vi "CJ_ADV.vi"() -> (5 "Plug in titles":string[](array[string]), 7 "Plug in values":string[](array[string]))   [LabVIEW 2010]
uses:
  Controls/Post_Process.ctl
  Globals/Meas_global.vi
  Globals/Plug_in_data_global.vi
panel:
  in  "Case Constant\n(See Context Help)":bool=TRUE
  out "Spectrum":cluster{dbl, dbl, dbl[][]}(graph)
  in  "Approx period":dbl=2.0 format="%.2f"
  in  "End chop":i32
  in  "Start chop":i32
  out "Auto correlation":cluster{dbl, dbl, dbl[]}[](graph)=[{0.2, 0.04, [0.46212378181095987, 0.44544943210747023, 0.39960558861098977, 0.3343117058776894, 0.2633632126098303, 0.21884653665959014, 0.1564325599910705, 0.12187113727101749, 0.06431157992181454, 0.0061376685707129775, -0.05669014852994204, -0.11505485081145915, -0.174459405708325, -0.19680472077091235, -0.2355643441337355, -0.279169576323247, -0.3107773861747396, -0.34177721677867895, -0.32552035787602773, -0.31390078612386346, -0.3141404513979377, -0.3203374677759062, -0.2805277493481923, -0.28030627175161327, -0.24878188504536167, -0.20171526154420918, -0.17478453331117821, -0.1492406112692455, -0.09716915086627186, -0.011036547249165897, 0.011273554688758552, 0.05137612064072646, 0.08633160095444244, 0.16325012318844126, 0.18825734545368525, 0.2399050524128652, 0.27148875410835505, 0.3135098324885922, 0.3339189753369369, 0.3532110595738442, 0.369889458228514, 0.4018515159612758, 0.3407037745996836, 0.3734587832352109, 0.33095796252280335, 0.3130223675527058, 0.28047256007652444, 0.2305017307249458, 0.24409104361634573, 0.22534283311709877, 0.19096120764523986, 0.10889483405727994, 0.06279838820183563, 0.014744937155805955, -0.02875404241397365, -0.02585905719816059, -0.06912125525736, -0.12596797235968518, -0.16959473872415834, -0.19587644981544367, -0.21534151184322906, -0.23255107675816336, -0.22831112695227931, -0.2179940037588913, -0.21577075545502555, -0.23768491590732238, -0.25009985440842564, -0.21883085511678074, -0.14982831467783184, -0.18257249609141823]}, {0.2, 0.04, [0.455531353534939, 0.4047541811650962, 0.3471922482149264, 0.2503699209196126, 0.20135079931123062, 0.11260724349217213, 0.034422569726896945, -0.030285571006114807, -0.11909404419991482, -0.18269038617194974, -0.23796709263127072, -0.2926953340047305, -0.35993422522198565, -0.4128421353811272, -0.45929580276986665, -0.5004541855522154, -0.5152391710086142, -0.51648559321319, -0.5271510882708651, -0.4806134161451423, -0.4850035395287815, -0.4662260004246924, -0.43183224812859133, -0.3975046428001596, -0.32639935049887153, -0.2795320771193606, -0.20861339510620014, -0.13136107527816313, -0.0788014018836706, -0.00855171247713191, 0.0298850880210123, 0.09776334527023417, 0.1785154642333505, 0.24021430276852615, 0.32501027179400727, 0.3418682226217491, 0.38756231445126293, 0.38959926105408205, 0.424467596341874, 0.4477619180529467, 0.4311914530598441, 0.4316664497716769, 0.4294595730219442, 0.4129090596655477, 0.3728855522699742, 0.35098699804248196, 0.3125013768615565, 0.25447334339580563, 0.20324298562375057, 0.166027641267823, 0.09557452943638053, 0.05023082102923798, -0.0032482398578684846, -0.05105953152757626, -0.13062652237796318, -0.19685300112362478, -0.24586301223225085, -0.2846838464872371, -0.3213134567643425, -0.3686474080102875, -0.40647088073256527, -0.4420878010421662, -0.4390774208886359, -0.4702929313038014, -0.4021180460569205, -0.37623488168286134, -0.3275070404289632, -0.3233751790837929, -0.2685900219122207, -0.23859579085375265]}]
  out "Clipped length":i32=524
  out "Time trace":cluster{dbl[], dbl[]}[](graph)
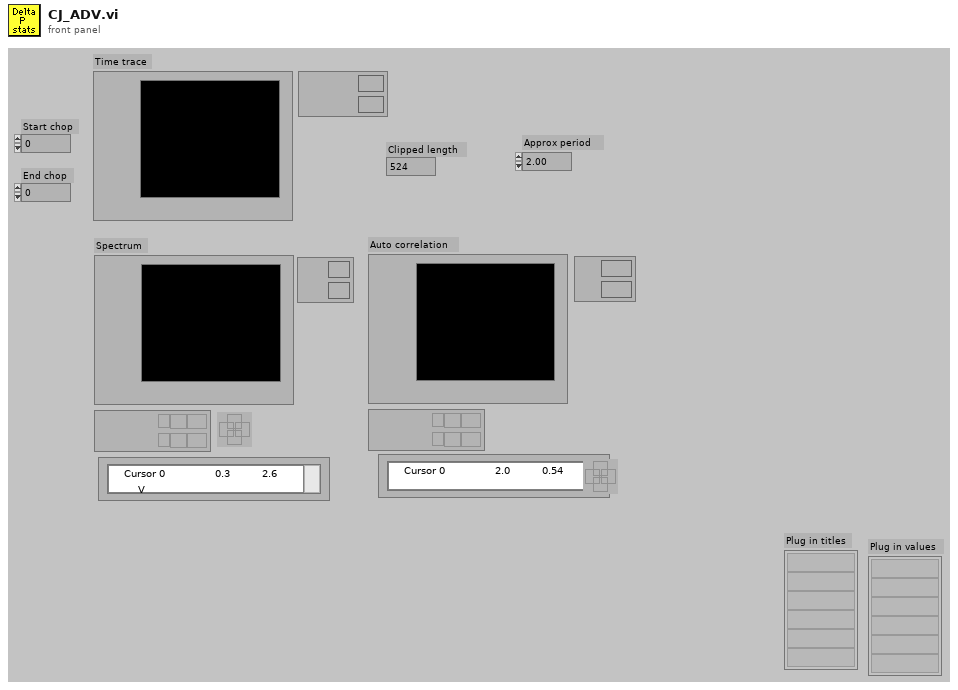
[diagram p1: front panel]
types:
  T1 = typedef "Post_Process.ctl" = enum16{"Take New Data", "Post Process Raw Data File"}
  T2 = typedef "Analysis_info_cluster.ctl" = cluster{"Colour":u32, "Inst type":T3, "Inst name":string, "Symbol":string, "Code name":string, "Extra Info":string, "Inst Array":T4, "Index":i32, "Voltage Index":i32, "Extra Titles":string[], "Extra Values":string[]}
  T3 = typedef "Inst_type.ctl" = enum16{"Propeller anemometer", "Raw voltage", "Pressure Transducer", "Pitot-static tube", "Preston tube", "Hot wire", "Cross wire 1", "Cross wire 2", "Generic Linear", "Generic Polynomial", "Generic BackPoly", "Fast FID", "Thermocouple", "Cold wire", "Pulsed Wire", "LDA Vel", "LDA Tran time", "LDA Arr time"}
  T4 = typedef "Instrument_Array.ctl" = enum16{"PWA", "LDA", "Analogue"}
  T5 = cluster{"Name":string, "X":dbl, "Y":dbl, "Z":dbl}[]
  T6 = cluster{"Name":string, "X":dbl, "Y":dbl, "Z":dbl}
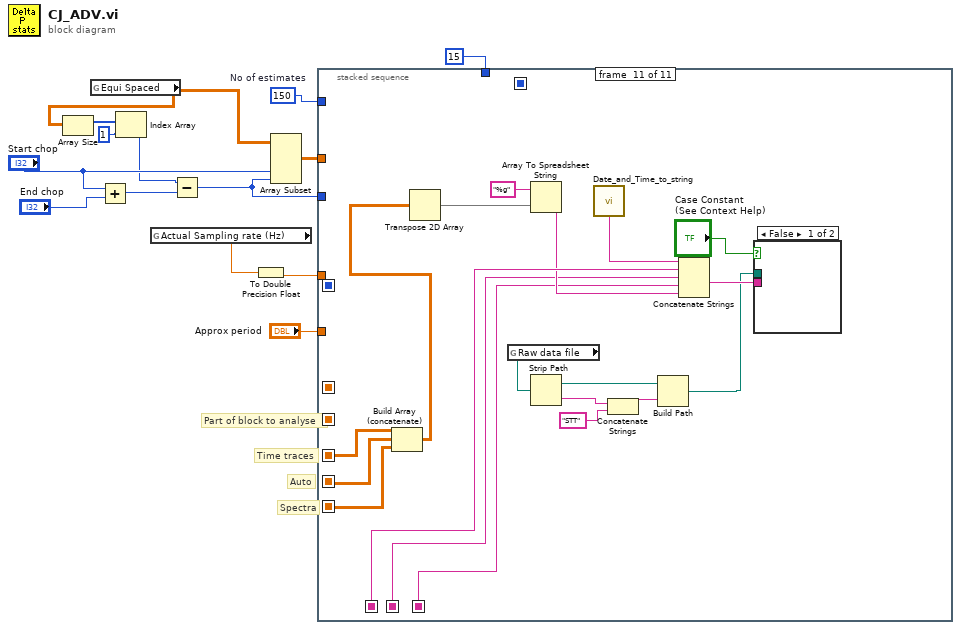
[diagram p0: block diagram]
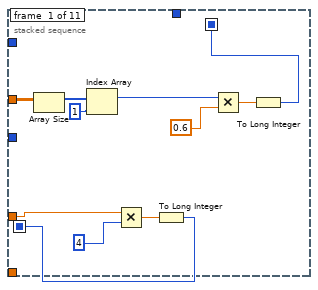
[diagram p2: hidden frame]
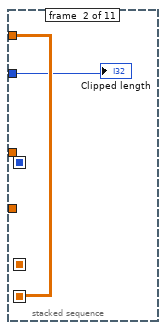
[diagram p3: hidden frame]
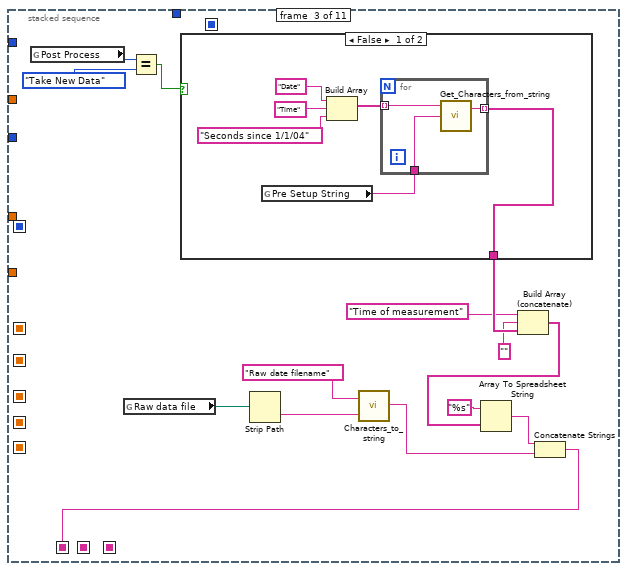
[diagram p4: hidden frame]
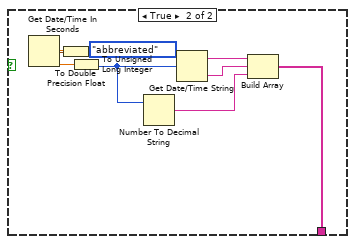
[diagram p5: hidden frame]
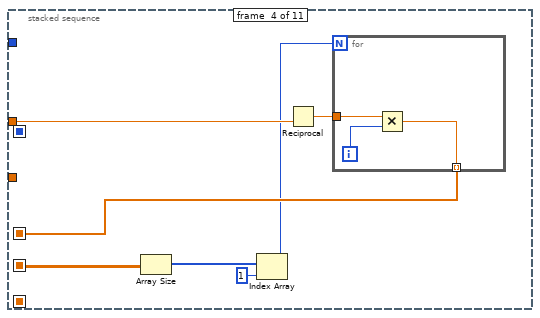
[diagram p6: hidden frame]
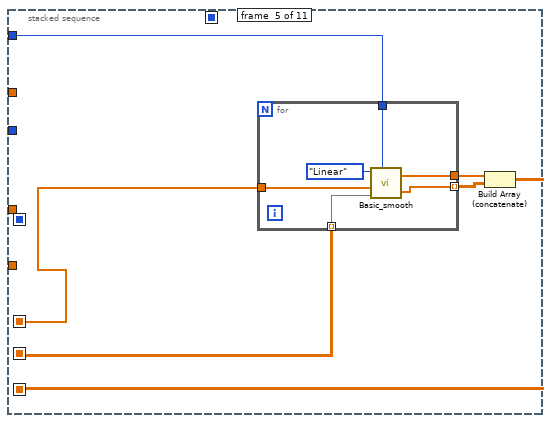
[diagram p7: hidden frame]
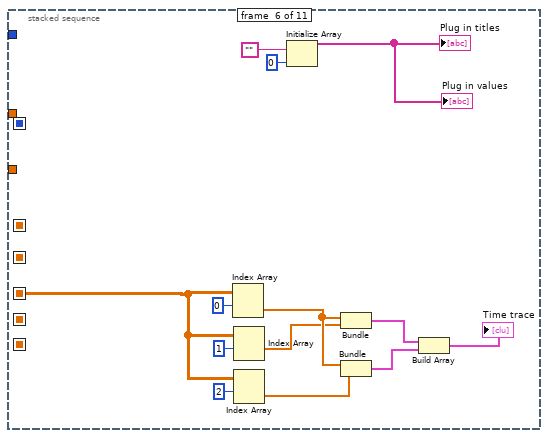
[diagram p8: hidden frame]
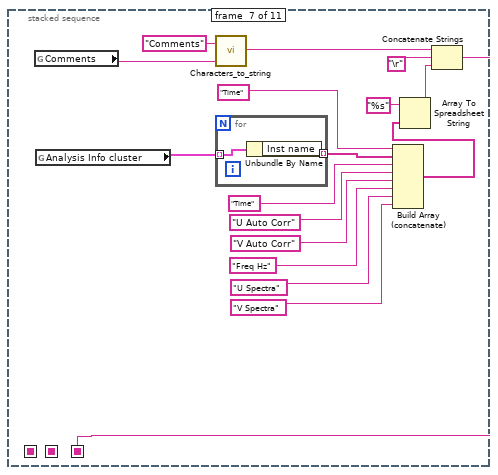
[diagram p9: hidden frame]
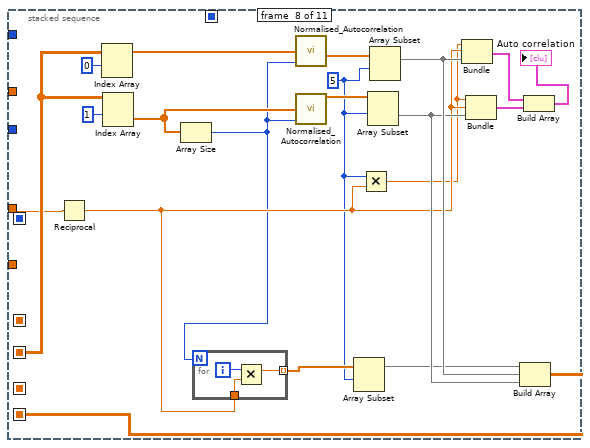
[diagram p10: hidden frame]
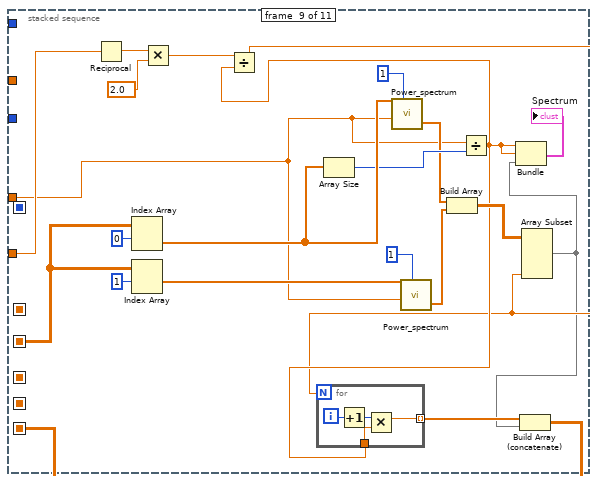
[diagram p11: hidden frame]
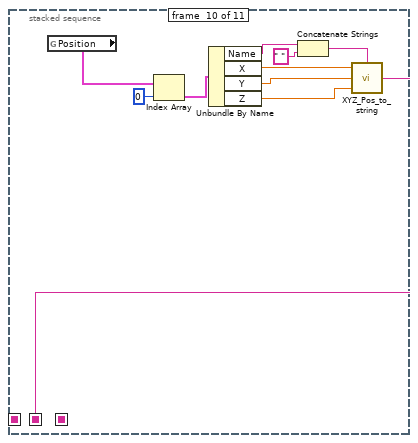
[diagram p12: hidden frame]
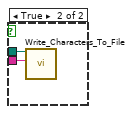
[diagram p13: hidden frame]
diagram:
  w14 = 150  # No of estimates
  # "Spectra"
  # "Auto"
  # "Part of block to analyse"
  # "Time traces"
  n1 = global read "Plug_in_data_global.vi" "Equi Spaced"() -> (w8:dbl[][])
  n2 = Array Size(array=w8) -> (size(s)=w9:i32[])
  n3 = Add(x="Start chop", y="End chop") -> (x+y=w4:i32)
  n4 = Index Array(array=w9, index=1) -> (element=w5:i32)
  n5 = global read "Meas_global.vi" "Actual Sampling rate (Hz)"() -> (w13:dbl)
  n6 = Subtract(x=w5, y=w4) -> (x-y=w1:i32)
  n7 = To Double Precision Float(number=w13) -> (double precision float=w12:dbl)
  n8 = Array Subset(array=w8, index (col)="Start chop", length (col)=w1) -> (w11:dbl[][])  [unwired: 2 in]
  n9 = stacked-sequence {
    seq-local: [_ _ _ _ _ _ w106 _ _ _ _] -> [_ _ _ _ _ _ _ _ _ _ w180]
    seq-local: [_ _ _ w64 _ _ _ _ _ _ _] -> [_ _ _ _ w74 _ _ _ _ _ _]
    seq-local: [_ _ _ _ w69 _ _ _ _ _ _] -> [_ _ _ _ _ w87 _ _ _ _ w185]
    seq-local: [_ _ w34 _ _ _ _ _ _ _ _] -> [_ _ _ _ _ _ _ _ _ _ w189]
    seq-local: [_ w27 _ _ _ _ _ _ _ _ _] -> [_ _ _ w60 w70 _ _ w128 w141 _ _]
    seq-local: [_ _ _ _ _ _ _ w125 _ _ _] -> [_ _ _ _ _ _ _ _ _ _ w184]
    seq-local: [_ _ _ _ _ _ _ _ _ w162 _] -> [_ _ _ _ _ _ _ _ _ _ w179]
    seq-local: [w16 _ _ _ _ _ _ _ _ _ _] -> [_ _ _ _ _ _ _ _ _ _ _]
    seq-local: [w15 _ _ _ _ _ _ _ _ _ _] -> [_ _ _ _ _ _ _ _ _ _ _]
    seq-local: [_ _ _ _ _ _ _ _ w136 _ _] -> [_ _ _ _ _ _ _ _ _ _ w178]
    tunnel: w12 -> [w18 _ _ w63 _ _ _ w124 w143 _ _]
    tunnel: w14 -> [_ _ _ _ w71 _ _ _ _ _ _]
    tunnel: w11 -> [w19 w27 _ _ _ _ _ _ _ _ _]
    tunnel: "Approx period" -> [_ _ _ _ _ _ _ _ w148 _ _]
    tunnel: 15 -> [_ _ _ _ _ _ _ _ _ _ _]
    tunnel: w1 -> [_ w26 _ _ _ _ _ _ _ _ _]
    frame #0 {
      n10 = Array Size(array=w19) -> (size(s)=w21:i32[])
      n11 = Index Array(array=w21, index=1) -> (element=w17:i32)
      n12 = Multiply(x=w18, y=4) -> (x*y=w24:dbl)
      n13 = To Long Integer(number=w24) -> (32bit integer=w15:i32)
      n14 = Multiply(x=w17, y=0.6) -> (x*y=w23:dbl)
      n15 = To Long Integer(number=w23) -> (32bit integer=w16:i32)
    }
    frame #1 {
      "Clipped length" <- w26
    }
    frame #2 {
      n16 = global read "Meas_global.vi" "Post Process"() -> (w40:T1)
      n17 = global read "Meas_global.vi" "Raw data file"() -> (w29:path)
      n18 = Equal?(x=w40, y=Post_Process."Take New Data" ("Post Process")) -> (x = y?=w39:bool)
      n19 = case shown="False" w39 {
        tunnel: [w42 w52] -> w33
        frame False {
          n20 = global read "Meas_global.vi" "Pre Setup String"() -> (w43:string)
          n21 = Build Array("Date", "Time", "Seconds since 1/1/04") -> (w44:string[])
          n22 = for {
            tunnel: w44 -> [w50] mode=indexing
            tunnel: w43 -> [w49]
            tunnel: [w48] -> w42 mode=indexing
            n23 = call "Get_Characters_from_string.vi"("Input string"=w49, "Variable name"=w50) -> ("Value"=w48:string)  [unwired: 1 in, 1 out]
          }
        }
        frame True {
          n24 = Get Date/Time In Seconds() -> (seconds since 1Jan1904=w51:timestamp)
          n25 = To Double Precision Float(number=w51) -> (double precision float=w55:dbl)
          n26 = To Unsigned Long Integer(number=w55) -> (unsigned 32bit integer=w54:u32)
          n27 = Number To Decimal String(number=w54) -> (decimal integer string=w53:string)  [unwired: 1 in]
          n28 = Get Date/Time String(date format (0)=enum16{"short", "long", "abbreviated"}."abbreviated", seconds (now)=w54) -> (date string=w57:string, time string=w56:string)  [unwired: 1 in]
          n29 = Build Array(w57, w56, w53) -> (w52:string[])
        }
      }
      n30 = Strip Path(path=w29) -> (name=w28:string)  [unwired: 1 out]
      n31 = call "Characters_to_string.vi"("Characters to write"=w28, "Label for characters"="Raw date filename") -> ("Output string"=w35:string)
      n32 = Build Array (concatenate)("Time of measurement", "" ("Value"), w33) -> (w30:string[])
      n33 = Array To Spreadsheet String(array=w30, 3:"%s" ("format string")) -> (spreadsheet string=w36:string)  [unwired: 1 in]
      n34 = Concatenate Strings(w36, w35) -> (w34:string)
    }
    frame #3 {
      n35 = Array Size(array=w60) -> (size(s)=w61:i32[])
      n36 = Index Array(array=w61, index=1) -> (element=w59:i32)
      n37 = Reciprocal(x=w63) -> (1/x=w65:dbl)
      n38 = for {
        N: w59 -> [_]
        tunnel: w65 -> [w68]
        tunnel: [w66] -> w64 mode=indexing
        i -> [w67]
        n39 = Multiply(x=w68, y=w67) -> (x*y=w66:dbl)
      }
    }
    frame #4 {
      n40 = for {
        tunnel: w74 -> [w79]
        tunnel: w70 -> [w78] mode=indexing
        tunnel: [w77] -> w73
        tunnel: [w76] -> w72 mode=indexing
        tunnel: w71 -> [w75]
        n41 = call "Basic_smooth.vi"("Smoothing"=enum16{"Linear", "Logarithmic"}."Linear", "X array in"=w79, "Y array in"=w78, "No of estimates output"=w75) -> ("X array Out"=w77:dbl[], "Y array Out"=w76:dbl[])  [unwired: 1 in]
      }
      n42 = Build Array (concatenate)(w73, w72) -> (w69:dbl[][])
    }
    frame #5 {
      n43 = Index Array(array=w87, index (row)=0) -> (element=w86:dbl[])  [unwired: 1 in]
      n44 = Index Array(array=w87, index (row)=1) -> (element=w81:dbl[])  [unwired: 1 in]
      n45 = Index Array(array=w87, index (row)=2) -> (element=w85:dbl[])  [unwired: 1 in]
      n46 = Initialize Array("", 0) -> (→"Plug in titles" →"Plug in values":string[])
      n47 = Bundle(w86, w81) -> (w84:cluster{dbl[], dbl[]})  [unwired: 1 in]
      n48 = Bundle(w86, w85) -> (w83:cluster{dbl[], dbl[]})  [unwired: 1 in]
      n49 = Build Array(w84, w83) -> (→"Time trace":cluster{dbl[], dbl[]}[])
    }
    frame #6 {
      n50 = global read "Meas_global.vi" "Comments"() -> (w110:string)
      n51 = global read "Meas_global.vi" "Analysis Info cluster"() -> (w105:T2[])
      n52 = call "Characters_to_string.vi"("Characters to write"=w110, "Label for characters"="Comments") -> ("Output string"=w108:string)
      n53 = for {
        tunnel: w105 -> [w112] mode=indexing
        tunnel: [w111] -> w104 mode=indexing
        n54 = Unbundle By Name(w112) -> ("Inst name"=w111:string)
      }
      n55 = Build Array (concatenate)("Time", w104, "Time", "U Auto Corr", "V Auto Corr", "Freq Hz", "U Spectra", "V Spectra") -> (w99:string[])
      n56 = Array To Spreadsheet String(array=w99, 3:"%s" ("format string")) -> (spreadsheet string=w98:string)  [unwired: 1 in]
      n57 = Concatenate Strings(w108, "\r", w98) -> (w106:string)
    }
    frame #7 {
      w116 = 5
      n58 = Reciprocal(x=w124) -> (1/x=w117:dbl)
      n59 = Index Array(array=w128, index (row)=0) -> (element=w129:dbl[])  [unwired: 1 in]
      n60 = Index Array(array=w128, index (row)=1) -> (element=w114:dbl[])  [unwired: 1 in]
      n61 = Array Size(array=w114) -> (size(s)=w113:i32)
      n62 = for {
        N: w113 -> [_]
        tunnel: w117 -> [w134]
        tunnel: [w133] -> w119 mode=indexing
        i -> [w135]
        n63 = Multiply(x=w135, y=w134) -> (x*y=w133:dbl)
      }
      n64 = call "Normalised_Autocorrelation.vi"("Autocorrelation length"=w113, "Array"=w129) -> ("Normalised Auto corr"=w123:dbl[])  [unwired: 1 in]
      n65 = call "Normalised_Autocorrelation.vi"("Autocorrelation length"=w113, "Array"=w114) -> ("Normalised Auto corr"=w122:dbl[])  [unwired: 1 in]
      n66 = Array Subset(array=w119, index=w116) -> (w118:dbl[])  [unwired: 1 in]
      n67 = Multiply(x=w116, y=w117) -> (x*y=w115:dbl)
      n68 = Array Subset(array=w122, index=w116) -> (w120:dbl[])  [unwired: 1 in]
      n69 = Array Subset(array=w123, index=w116) -> (w121:dbl[])  [unwired: 1 in]
      n70 = Bundle(w115, w117, w121) -> (w127:cluster{dbl, dbl, dbl[]})  [unwired: 1 in]
      n71 = Bundle(w115, w117, w120) -> (w126:cluster{dbl, dbl, dbl[]})  [unwired: 1 in]
      n72 = Build Array(w118, w121, w120) -> (w125:dbl[][])
      n73 = Build Array(w127, w126) -> (→"Auto correlation":cluster{dbl, dbl, dbl[]}[])
    }
    frame #8 {
      n74 = Reciprocal(x=w148) -> (1/x=w147:dbl)
      n75 = Index Array(array=w141, index (row)=0) -> (element=w154:dbl[])  [unwired: 1 in]
      n76 = Index Array(array=w141, index (row)=1) -> (element=w151:dbl[])  [unwired: 1 in]
      n77 = Multiply(x=w147, y=2.0) -> (x*y=w145:dbl)
      n78 = Array Size(array=w154) -> (size(s)=w153:i32)
      n79 = call "Power_spectrum.vi"("U"=w154, "Sampling frequency"=w143, "Block No"=1) -> ("Spectrum output array"=w150:dbl[])  [unwired: 3 in]
      n80 = call "Power_spectrum.vi"("U"=w151, "Sampling frequency"=w143, "Block No"=1) -> ("Spectrum output array"=w149:dbl[])  [unwired: 3 in]
      n81 = Build Array(w150, w149) -> (w144:dbl[][])
      n82 = Divide(x=w143, y=w153) -> (x/y=w140:dbl)
      n83 = Divide(x=w145, y=w140) -> (x/y=w139:dbl)
      n84 = for {
        N: w139 -> [_]
        tunnel: w140 -> [w160]
        tunnel: [w158] -> w138 mode=indexing
        i -> [w161]
        n85 = Increment(x=w161) -> (x+1=w159:i32)
        n86 = Multiply(x=w159, y=w160) -> (x*y=w158:dbl)
      }
      n87 = Array Subset(array=w144, length (col)=w139) -> (w137:dbl[][])  [unwired: 3 in]
      n88 = Bundle(w140, w140, w137) -> (→"Spectrum":cluster{dbl, dbl, dbl[][]})  [unwired: 1 in]
      n89 = Build Array (concatenate)(w138, w137) -> (w136:dbl[][])
    }
    frame #9 {
      n90 = global read "Meas_global.vi" "Position"() -> (w163:T5)
      n91 = Index Array(array=w163, index=0) -> (element=w170:T6)
      n92 = Unbundle By Name(w170) -> ("Name"=w164:string, "X"=w168:dbl, "Y"=w167:dbl, "Z"=w166:dbl)
      n93 = Concatenate Strings(w164, " " ("Output string")) -> (w169:string)
      n94 = call "XYZ_Pos_to_string.vi"("Position label"=w169, "Z"=w166, "Y"=w167, "X"=w168) -> ("Output string"=w162:string)
    }
    frame #10 {
      n95 = Build Array (concatenate)(w185, w184, w178) -> (w182:dbl[][])
      n96 = Transpose 2D Array(2D array=w182) -> (transposed array=w190:dbl[][])
      n97 = global read "Meas_global.vi" "Raw data file"() -> (w176:path)
      n98 = Array To Spreadsheet String(array=w190, 3:"%g" ("format string")) -> (spreadsheet string=w181:string)  [unwired: 1 in]
      n99 = Strip Path(path=w176) -> (stripped path=w173:path, name=w175:string)
      n100 = call "Date_and_Time_to_string.vi"() -> ("Date and time (spreadsheet)"=w183:string)
      n101 = Concatenate Strings(w175, "STT") -> (w174:string)
      n102 = Build Path(base path=w173, name or relative path=w174) -> (appended path=w172:path)
      n103 = Concatenate Strings(w183, w189, w179, w180, w181) -> (w187:string)
      n104 = case shown="False" "Case Constant\n(See Context Help)" {
        tunnel: w187 -> [_ w192]
        tunnel: w172 -> [_ w191]
        frame False {
        }
        frame True {
          n105 = call "Write_Characters_To_File.vi"("file path (dialog if empty)"=w191, "character string"=w192) -> ()  [unwired: 6 in, 1 out]
        }
      }
    }
  }
